vi "StaticWrite.vi"(8 "error in (no error)":errorcluster, 9 "StaticValue":dbl, 10 "Channel":u8, 11 "AIO in":refnum<class "AIO.lvclass">) -> (0 "error out":errorcluster, 3 "AIO out":refnum<class "AIO.lvclass">)   [LabVIEW 2024, in "AIO Actor.lvlib" / "AIO.lvclass"]
uses:
  AIO.lvclass
  AO Type.ctl
  AIO.lvclass/AIO.ctl
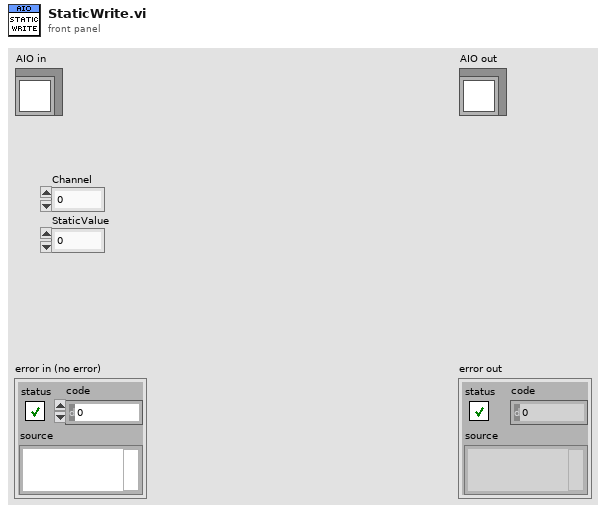
[diagram p1: front panel]
types:
  T1 = typedef "AO Type.ctl" = enum16{"Static", "Streaming", "StopStreaming"}
  T2 = cluster{"AoType":T1, "Channel":u8, "StaticValue":dbl, "WavePara":cluster{"Crest":dbl, "Trough":dbl, "Period":dbl}}
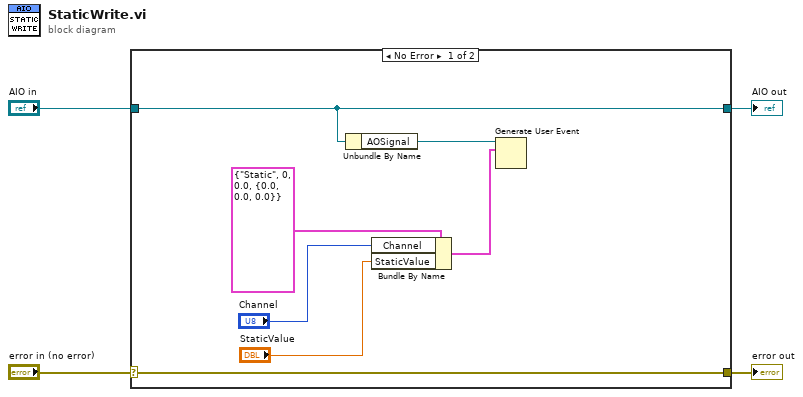
[diagram p0: block diagram]
diagram:
  n1 = case shown="No Error" "error in (no error)" {
    selector: "error in (no error)" -> [w11 w13]
    tunnel: [w11 w13] -> w3
    tunnel: [w10 w12] -> w1
    tunnel: "AIO in" -> [w10 w12]
    frame No Error {
      n2 = Unbundle By Name(w10) -> ("AOSignal"=w9:refnum<user-event>)
      n3 = Bundle By Name(cluster=T2 {"AoType"=enum."Static", "Channel"=0, "StaticValue"=0.0, "WavePara"={"Crest"=0.0, "Trough"=0.0, "Period"=0.0}} ("event data"), "Channel"="Channel", "StaticValue"="StaticValue") -> (w5:T2)
      n4 = Generate User Event(user event=w9, event data cluster=w5) -> ()  [unwired: 2 in, 2 out]
    }
    frame Error {
    }
  }
  "error out" <- w3
  "AIO out" <- w1
